vi "Control Variant Values to Double Values.vi"(6 "class names":string, 8 "error in (no error)":errorcluster, 9 "variant values":variant) -> (0 "error out":errorcluster, 1 "values":dbl)   [LabVIEW 2020]
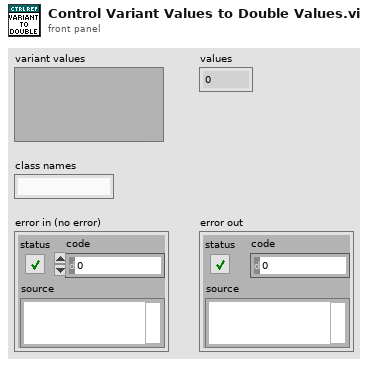
[diagram p1: front panel]
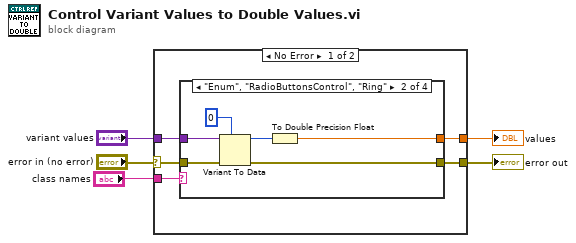
[diagram p0: block diagram]
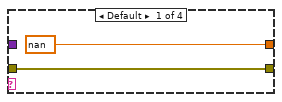
[diagram p2: hidden frame]
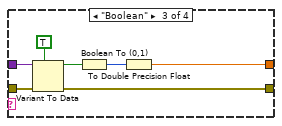
[diagram p3: hidden frame]
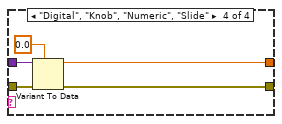
[diagram p4: hidden frame]
diagram:
  n1 = case shown="No Error" "error in (no error)" {
    selector: "error in (no error)" -> [w6 w31]
    tunnel: "class names" -> [w10 _]
    tunnel: "variant values" -> [w9 _]
    tunnel: [w8 _] -> w3
    tunnel: [w7 w31] -> w2
    frame No Error {
      n2 = case shown="\"Enum\", \"RadioButtonsControl\", \"Ring\"" w10 {
        tunnel: w6 -> [w12 w18 w25 w30]
        tunnel: [nan w13 w21 w26] -> w8
        tunnel: [w12 w17 w24 w29] -> w7
        tunnel: w9 -> [_ w16 w23 w28]
        frame Default {
        }
        frame "Enum", "RadioButtonsControl", "Ring" {
          n3 = Variant To Data(error in=w18, type=0, Variant=w16) -> (data=w14:i32, error out=w17:errorcluster)
          n4 = To Double Precision Float(number=w14) -> (double precision float=w13:dbl)
        }
        frame "Boolean" {
          n5 = Variant To Data(error in=w25, type=TRUE, Variant=w23) -> (data=w20:bool, error out=w24:errorcluster)
          n6 = Boolean To (0,1)(Boolean=w20) -> (0, 1=w19:i16)
          n7 = To Double Precision Float(number=w19) -> (double precision float=w21:dbl)
        }
        frame "Digital", "Knob", "Numeric", "Slide" {
          n8 = Variant To Data(error in=w30, type=0.0, Variant=w28) -> (data=w26:dbl, error out=w29:errorcluster)
        }
      }
    }
    frame Error {
    }
  }
  "values" <- w3
  "error out" <- w2
